vi "例8.11-2利用DAQmx函数连续输出正弦波且参数可调.vi"() -> ()   [LabVIEW 2017]
uses:
  <vilib>/DAQmx/write.llb/DAQmx Write (Analog Wfm 1Chan NSamp).vi
  <vilib>/DAQmx/create/channels.llb/DAQmx Create Channel (AO-Voltage-Basic).vi
  <vilib>/DAQmx/configure/timing.llb/DAQmx Timing (Sample Clock).vi
  <vilib>/DAQmx/miscellaneous.llb/DAQmx Fill In Error Info.vi
  <vilib>/measure/NI_MABase.lvlib
  <resource>/objmgr/daqmx.rc
panel:
  out "采集卡的采样率":dbl
  in  "amplitude":dbl=1.0 caption="幅值" format="%0.2p"
  in  "frequency":dbl=10.0 caption="频率" format="%0.2p"
  out "波形图":waveform(dbl)(graph)
  in  "停止":bool
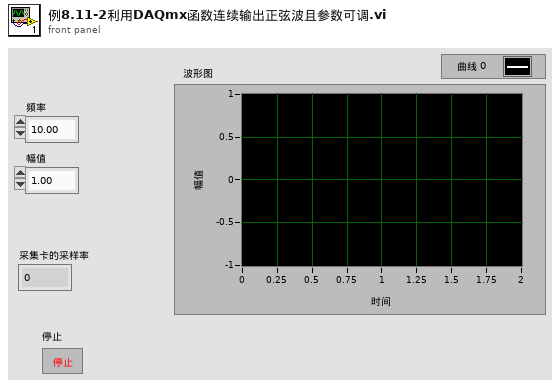
[diagram p1: front panel]
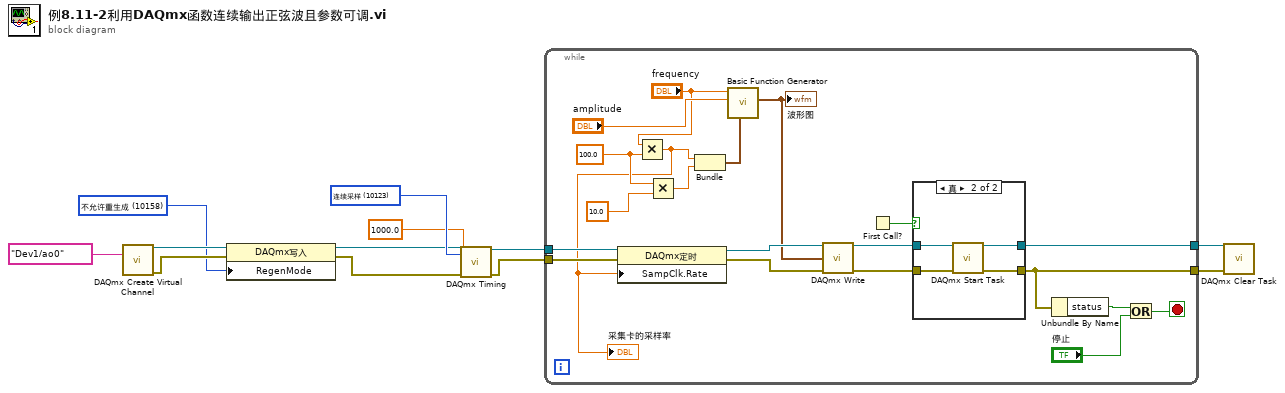
[diagram p0: block diagram]
diagram:
  w5 = 10158 items=["允许重生成"=10097, "不允许重生成"=10158] ("RegenMode")
  w11 = 10123 items=["有限采样"=10178, "连续采样"=10123, "硬件定时单点"=12522] ("sample mode")
  n1 = call-poly <vilib>:"DAQmx Create Virtual Channel.vi"("physical channels"=tag "Dev1/ao0") -> ("task out"=w9:refnum<k21>, "error out"=w8:errorcluster)  [unwired: 13 in]
  n2 = property class="DAQmx写入"(reference=w9, error in=w8, "RegenMode"=w5) -> (reference out=w7:refnum<k21>, error out=w6:errorcluster)
  n3 = call-poly <vilib>:"DAQmx Timing.vi"("task/channels in"=w7, "sample mode"=w11, "rate"=1000.0, "error in"=w6) -> ("task out"=w4:refnum<k21>, "error out"=w3:errorcluster)  [unwired: 10 in]
  n4 = while {
    tunnel: w4 -> [w26]
    tunnel: w3 -> [w25]
    tunnel: [w16] -> w2
    tunnel: [w14] -> w1
    stop <- w13 stop-if-true
    w30 = 100.0 ("y")
    n5 = Multiply(x="frequency", y=w30) -> (x*y=w23:dbl)
    "采集卡的采样率" <- w23
    n6 = property class="DAQmx定时"(reference=w26, error in=w25, "SampClk.Rate"=w23) -> (reference out=w22:refnum<k21>, error out=w21:errorcluster)
    n7 = Multiply(x=w30, y=10.0) -> (x*y=w28:dbl)
    n8 = Bundle(w23, w28) -> (w27:cluster{dbl, dbl})  [unwired: 1 in]
    n9 = call <vilib>:"Basic Function Generator.vi"("sampling info"=w27, "amplitude"="amplitude", "frequency"="frequency") -> ("signal out"=w20:waveform(dbl))  [unwired: 6 in, 2 out]
    "波形图" <- w20
    n10 = call-poly <vilib>:"DAQmx Write.vi"("task/channels in"=w22, "data"=w20, "error in"=w21) -> ("task out"=w18:refnum<k21>, "error out"=w17:errorcluster)  [unwired: 10 in, 1 out]
    n11 = First Call?() -> (First Call?: T/F=w19:bool)
    n12 = case shown="真" w19 {
      tunnel: w18 -> [w34 w38]
      tunnel: w17 -> [w33 w37]
      tunnel: [w34 w36] -> w16
      tunnel: [w33 w35] -> w14
      frame False {
      }
      frame True {
        n13 = call <vilib>:"DAQmx Start Task.vi"("task/channels in"=w38, "error in"=w37) -> ("task out"=w36:refnum<k21>, "error out"=w35:errorcluster)  [unwired: 12 in]
      }
    }
    n14 = Unbundle By Name(w14) -> ("status"=w15:bool)
    n15 = Or(x=w15, y="停止") -> (x .or. y?=w13:bool)
  }
  n16 = call <vilib>:"DAQmx Clear Task.vi"("task in"=w2, "error in"=w1) -> ()  [unwired: 13 in, 1 out]
